vi "Sort2D.vi"(3 "Transpose":bool=TRUE, 4 "2D array to sort":dbl[][](array[numeric]) format="%.2f", 5 "Descending":bool) -> (1 "Sorted array":dbl[][](array[numeric]) format="%.2f")   [LabVIEW 2013]
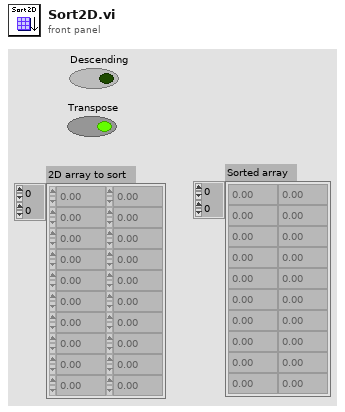
[diagram p1: front panel]
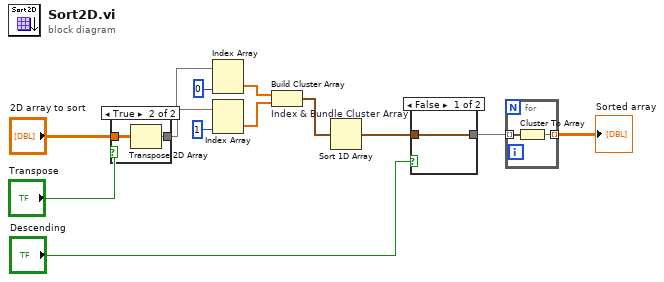
[diagram p0: block diagram]
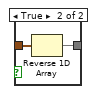
[diagram p2: hidden frame]
diagram:
  n1 = case shown="True" "Transpose" {
    tunnel: "2D array to sort" -> [w13 w15]
    tunnel: [w13 w14] -> w4
    frame False {
    }
    frame True {
      n2 = Transpose 2D Array(2D array=w15) -> (transposed array=w14:dbl[][])
    }
  }
  n3 = Index Array(array=w4, index (col)=0) -> (element=w12:dbl[])  [unwired: 1 in]
  n4 = Index Array(array=w4, index (col)=1) -> (element=w11:dbl[])  [unwired: 1 in]
  n5 = Build Cluster Array "Index & Bundle Cluster Array"(w12, w11) -> (w10:cluster{dbl, dbl}[])
  n6 = Sort 1D Array(array=w10) -> (sorted array=w9:cluster{dbl, dbl}[])
  n7 = case shown="False" "Descending" {
    tunnel: w9 -> [w16 w18]
    tunnel: [w16 w17] -> w2
    frame False {
    }
    frame True {
      n8 = Reverse 1D Array(array=w18) -> (reversed array=w17:cluster{dbl, dbl}[])
    }
  }
  n9 = for {
    tunnel: w2 -> [w20] mode=indexing
    tunnel: [w19] -> w8 mode=indexing
    n10 = Cluster To Array(cluster=w20) -> (array=w19:dbl[])
  }
  "Sorted array" <- w8
